vi "Log Data.vi"(7 "Command":enum16{"Initialize", "Write", "Stop"}(ring), 8 "error in (no error)":errorcluster, 10 "Event Data":string[](array[string]), 11 "file path":path) -> (0 "error out":errorcluster)   [LabVIEW 2013]
uses:
  <vilib>/Utility/file.llb/Write To Spreadsheet File (string).vi
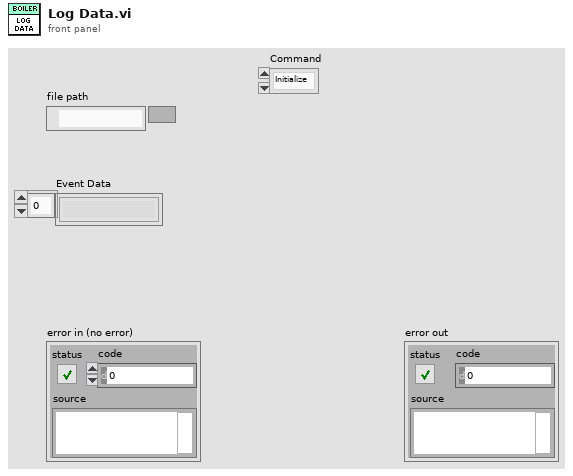
[diagram p1: front panel]
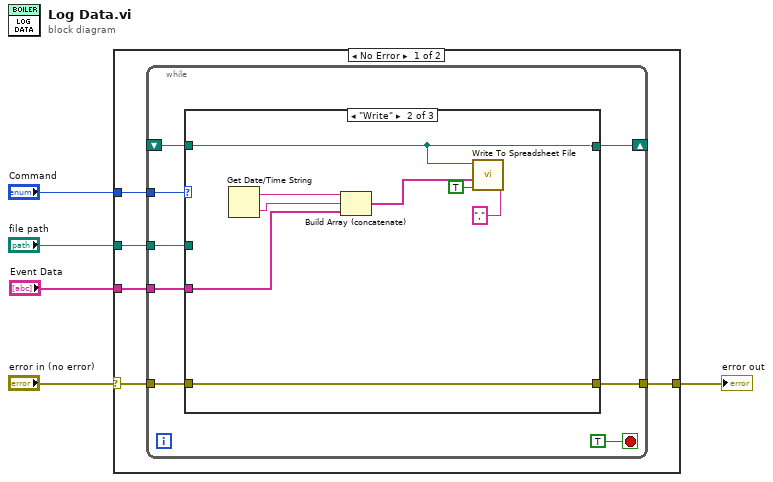
[diagram p0: block diagram]
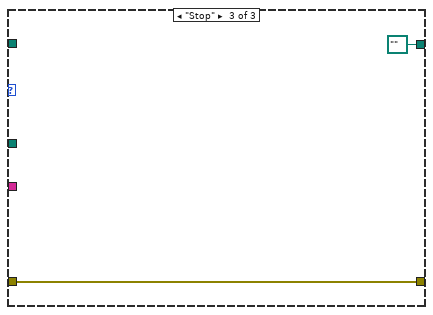
[diagram p3: hidden frame]
diagram:
  n1 = case shown="No Error" "error in (no error)" {
    selector: "error in (no error)" -> [w8 w31]
    tunnel: "Command" -> [w10 _]
    tunnel: "file path" -> [w9 _]
    tunnel: [w7 w31] -> w5
    tunnel: "Event Data" -> [w6 _]
    frame No Error {
      n2 = while {
        tunnel: w10 -> [w18]
        tunnel: w9 -> [w17]
        shift-right: [w16] -> _
        shift-left: _ -> [w15]
        tunnel: w8 -> [w14]
        tunnel: [w13] -> w7
        tunnel: w6 -> [w12]
        stop <- TRUE stop-if-true
        n3 = case shown="\"Write\"" w18 {
          tunnel: w17 -> [w20 _ _]
          tunnel: [w20 w28 path "" ("file path")] -> w16
          tunnel: w15 -> [_ w28 _]
          tunnel: w14 -> [w19 w25 w29]
          tunnel: [w19 w25 w29] -> w13
          tunnel: w12 -> [_ w24 _]
          frame "Initialize", Default {
          }
          frame "Write" {
            n4 = Get Date/Time String() -> (date string=w27:string, time string=w26:string)  [unwired: 3 in]
            n5 = Build Array (concatenate)(w27, w26, w24) -> (w22:string[])
            n6 = call-poly <vilib>:"Write To Spreadsheet File.vi"("delimiter (\\t)"="," ("delimiter (\\t)"), "append to file? (new file:F)"=TRUE, "1D data"=w22, "file path (dialog if empty)"=w28) -> ()  [unwired: 4 in, 1 out]
          }
          frame "Stop" {
          }
        }
      }
    }
    frame Error {
    }
  }
  "error out" <- w5
